vi "ACQUIRE.vi"() -> ()   [LabVIEW 2013]
uses:
  Global.vi
panel:
  out "error out":errorcluster
  in  "stop":bool
  out "VAR index":i32
  out "Val":dbl=4000.0 format="%.2f"
  in  "Old_Val":dbl=4000.0
  out "Set":bool
  out "Recieved":bool
  in  "Var":string="ACQ"
  # "Sets the acquisition time (s)\nof sequencer.vi.\n\nValue Type: I32\nOptions: None"
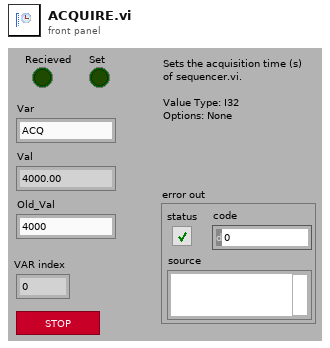
[diagram p1: front panel]
types:
  T1 = typedef "Semaphore RefNum" = refnum<k1>
  T2 = cluster{"VAR":string, "Options":string, "Val":string, "Recieved":bool, "Set":bool}[]
  T3 = cluster{"VAR":string, "Options":string, "Val":string, "Recieved":bool, "Set":bool}
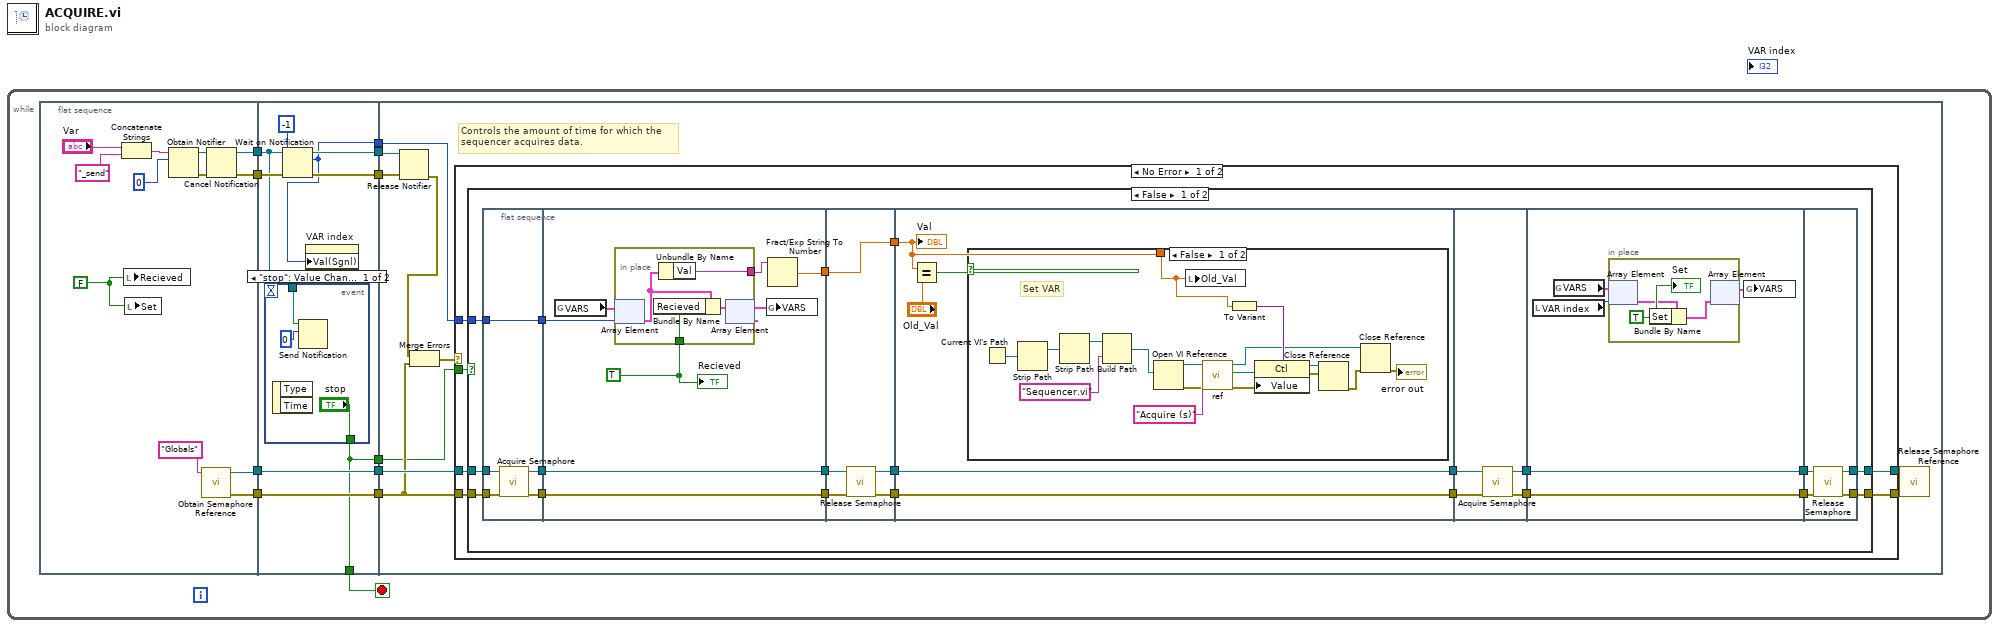
[diagram p0: block diagram]
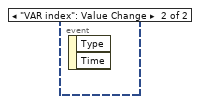
[diagram p2: hidden frame]
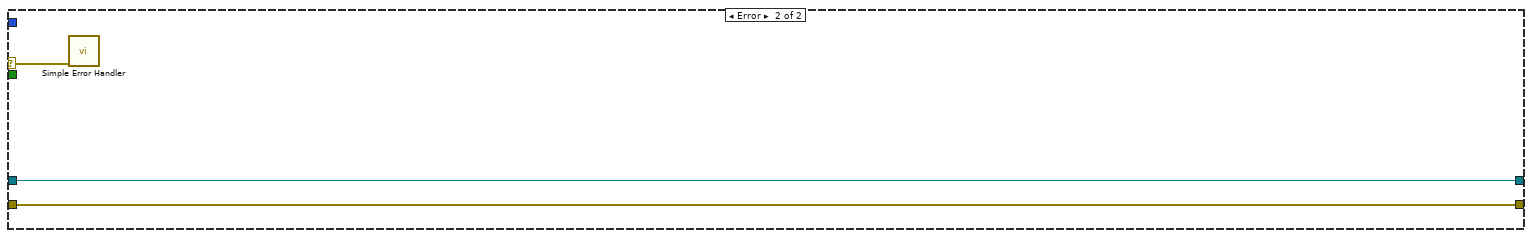
[diagram p5: hidden frame]
diagram:
  n1 = while {
    stop <- w2 stop-if-true
    n2 = flat-sequence {
      tunnel: [w14] -> w11
      tunnel: [w13] -> w10
      tunnel: [w21] -> w6
      tunnel: [w20] -> w4
      tunnel: w11 -> [w31]
      tunnel: w10 -> [w25]
      tunnel: [w30] -> w9
      tunnel: [w27] -> w8
      tunnel: [w26] -> w7
      tunnel: w6 -> [w29]
      tunnel: [w29] -> w5
      tunnel: w4 -> [w28]
      tunnel: [w28] -> w3
      tunnel: [w24] -> w2
      tunnel: [w24] -> w1
      tunnel: w9 -> [w38]
      tunnel: w8 -> [w39]
      tunnel: w7 -> [w45]
      tunnel: w5 -> [w44]
      tunnel: w3 -> [w41]
      tunnel: w1 -> [w36]
      frame #0 {
        w23 = FALSE ("notification")
        n3 = Concatenate Strings("Var", "_send") -> (w18:string)
        n4 = local write "Recieved"(w23) -> ()
        n5 = local write "Set"(w23) -> ()
        n6 = Obtain Notifier(name (unnamed)=w18, notification data type=0) -> (notifier out=w12:refnum<notifier>, error out=w15:errorcluster)  [unwired: 2 in, 1 out]
        n7 = call <vilib>:"Obtain Semaphore Reference.vi"("name (unnamed)"="Globals") -> ("error out"=w20:errorcluster, "semaphore"=w21:T1)  [unwired: 4 in, 1 out]
        n8 = Cancel Notification(0:w12, 3:w15) -> (8:w13:refnum<notifier>, 11:w14:errorcluster)  [unwired: 1 out]
      }
      frame #1 {
        n9 = event shown="[0] \"stop\": Value Change" {
          selector: _ -> [_ _]
          dyn-events: _ -> [_ _]
          timeout: _ -> [_ _]
          tunnel: ["stop" _] -> w24
          tunnel: w25 -> [w34 _]
          event "stop": Value Change {
            n10 = event-data() -> ()  [unwired: 1 in, 2 out]
            n11 = Send Notification(notification=0, notifier=w34) -> ()  [unwired: 1 in, 2 out]
          }
          event "VAR index": Value Change {
            n12 = event-data() -> ()  [unwired: 1 in, 2 out]
          }
        }
        n13 = Wait on Notification(notifier=w25, timeout in ms (-1)=-1, error in (no error)=w31) -> (notifier out=w30:refnum<notifier>, notification=w26:i32, error out=w27:errorcluster)  [unwired: 1 in, 1 out]
        n14 = property on="VAR index" class="DigNum (strict)"("Val(Sgnl)"=w26) -> ()  [unwired: 2 in, 2 out]
      }
      frame #2 {
        # "Controls the amount of time for which the \nsequencer acquires data."
        n15 = Release Notifier(notifier=w38, error in (no error)=w39) -> (error out=w37:errorcluster)  [unwired: 1 in, 2 out]
        n16 = Merge Errors(w37, w41) -> (w40:errorcluster)
        n17 = case shown="No Error" w40 {
          selector: w40 -> [_ w134]
          tunnel: w45 -> [w51 _]
          tunnel: w44 -> [w50 w136]
          tunnel: w41 -> [w49 w135]
          tunnel: [w48 w135] -> w43
          tunnel: [w47 w136] -> w42
          tunnel: w36 -> [w46 _]
          frame No Error {
            n18 = case shown="False" w46 {
              tunnel: w51 -> [w56 _]
              tunnel: w50 -> [w55 w133]
              tunnel: w49 -> [w54 w132]
              tunnel: [w53 w132] -> w48
              tunnel: [w52 w133] -> w47
              frame False {
                n19 = flat-sequence {
                  tunnel: w54 -> [w74]
                  tunnel: w55 -> [w75]
                  tunnel: w56 -> [w76]
                  tunnel: [w76] -> w71
                  tunnel: [w73] -> w70
                  tunnel: [w72] -> w69
                  tunnel: w71 -> [w79]
                  tunnel: w70 -> [w83]
                  tunnel: w69 -> [w84]
                  tunnel: [w84] -> w68
                  tunnel: [w83] -> w67
                  tunnel: [w77] -> w66
                  tunnel: w68 -> [w92]
                  tunnel: w67 -> [w93]
                  tunnel: [w91] -> w65
                  tunnel: [w90] -> w64
                  tunnel: [w89] -> w63
                  tunnel: w66 -> [w89]
                  tunnel: w65 -> [w97]
                  tunnel: w64 -> [w96]
                  tunnel: [w97] -> w62
                  tunnel: [w96] -> w61
                  tunnel: w63 -> [w94]
                  tunnel: w62 -> [w119]
                  tunnel: w61 -> [w116]
                  tunnel: [w118] -> w60
                  tunnel: [w117] -> w59
                  tunnel: [w124] -> w58
                  tunnel: w60 -> [w124]
                  tunnel: [w120] -> w57
                  tunnel: w59 -> [w120]
                  tunnel: w58 -> [w131]
                  tunnel: w57 -> [w130]
                  tunnel: [w129] -> w53
                  tunnel: [w128] -> w52
                  frame #0 {
                    n20 = call <vilib>:"Acquire Semaphore.vi"("error in (no error)"=w74, "semaphore"=w75) -> ("error out"=w73:errorcluster, "semaphore out"=w72:T1)  [unwired: 3 in, 1 out]
                  }
                  frame #1 {
                    w80 = TRUE ("Found")
                    n21 = global read "Global.vi" "VARS"() -> (w81:T2)
                    n22 = in-place {
                      in-place-border: [w86] -> w78
                      in-place-border: w80 -> [w85]
                      n23 = in-place-array #1(w81, w79) -> (w88:T3)
                      n24 = Bundle By Name(cluster=w88, "Recieved"=w85) -> (w87:T3)
                      n25 = Unbundle By Name(w88) -> ("Val"=w86:string)
                      n26 = in-place-array #1(w87) -> (w82:T2)  [unwired: 1 out]
                    }
                    n27 = global write "Global.vi" "VARS"(w82) -> ()
                    n28 = Fract/Exp String To Number(string=w78) -> (number=w77:dbl)  [unwired: 3 in, 1 out]
                    "Recieved" <- w80
                  }
                  frame #2 {
                    n29 = call <vilib>:"Release Semaphore.vi"("error in (no error)"=w93, "semaphore"=w92) -> ("error out"=w90:errorcluster, "semaphore out"=w91:T1)  [unwired: 4 in]
                  }
                  frame #3 {
                    n30 = Equal?(x=w94, y="Old_Val") -> (x = y?=w95:bool)
                    n31 = case shown="False" w95 {
                      tunnel: w94 -> [w113 _]
                      frame False {
                        # "Set VAR"
                        n32 = Current VI's Path() -> (path=w100:path)
                        n33 = Strip Path(path=w100) -> (stripped path=w101:path)  [unwired: 1 out]
                        n34 = Strip Path(path=w101) -> (stripped path=w102:path)  [unwired: 1 out]
                        n35 = Build Path(base path=w102, name or relative path="Sequencer.vi") -> (appended path=w99:path)
                        n36 = Open VI Reference(vi path=w99) -> (vi reference=w105:refnum<vi>, error out=w104:errorcluster)  [unwired: 5 in]
                        n37 = local write "Old_Val"(w113) -> ()
                        n38 = call "ref.vi"("error in (no error)"=w104, "Name"="Acquire (s)", "VI reference"=w105) -> ("error out"=w111:errorcluster, "Ctrl reference out"=w114:refnum<vi>, "VI reference out"=w106:refnum<vi>)  [unwired: 5 in, 1 out]
                        n39 = To Variant(anything=w113) -> (Variant=w112:variant)
                        n40 = property class="Ctl"(reference=w114, error in=w111, "Value"=w112) -> (reference out=w110:refnum<vi>, error out=w109:errorcluster)
                        n41 = Close Reference(reference=w110, error in (no error)=w109) -> (error out=w108:errorcluster)
                        n42 = Close Reference(reference=w106, error in (no error)=w108) -> (error out=→"error out":errorcluster)
                      }
                      frame True {
                      }
                    }
                    "Val" <- w94
                  }
                  frame #4 {
                    n43 = call <vilib>:"Acquire Semaphore.vi"("error in (no error)"=w116, "semaphore"=w119) -> ("error out"=w117:errorcluster, "semaphore out"=w118:T1)  [unwired: 3 in, 1 out]
                  }
                  frame #5 {
                    n44 = local read "VAR index"() -> (w123:i32)
                    n45 = global read "Global.vi" "VARS"() -> (w122:T2)
                    n46 = in-place {
                      w127 = TRUE ("Set")
                      n47 = in-place-array #2(w122, w123) -> (w126:T3)
                      n48 = Bundle By Name(cluster=w126, "Set"=w127) -> (w125:T3)
                      n49 = in-place-array #2(w125) -> (w121:T2)  [unwired: 1 out]
                      "Set" <- w127
                    }
                    n50 = global write "Global.vi" "VARS"(w121) -> ()
                  }
                  frame #6 {
                    n51 = call <vilib>:"Release Semaphore.vi"("error in (no error)"=w130, "semaphore"=w131) -> ("error out"=w129:errorcluster, "semaphore out"=w128:T1)  [unwired: 4 in]
                  }
                }
              }
              frame True {
              }
            }
          }
          frame Error {
            n52 = call <vilib>:"Simple Error Handler.vi"("error in (no error)"=w134) -> ()  [unwired: 4 in, 5 out]
          }
        }
        n53 = call <vilib>:"Release Semaphore Reference.vi"("error in (no error)"=w43, "semaphore"=w42) -> ()  [unwired: 8 in, 2 out]
      }
    }
  }
